vi "Async Test.vi"(11 "gRPCid":T1) -> ()   [LabVIEW 2019]
uses:
  ScanList/labview-grpc-query-server/VIs/MeasurementServer_gRPCid.ctl
  ScanList/labview-grpc-query-server/VIs/MeasurementServer_ErrorOutData.ctl
  ScanList/labview-grpc-query-server/VIs/MeasurementServer_FourProbeRawData.ctl
  ScanList/labview-grpc-query-server/VIs/labview-grpc-measurement-server.lvlib
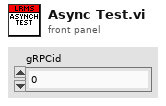
[diagram p1: front panel]
types:
  T1 = typedef "labview-grpc-measurement-server.lvlib/MeasurementServer_gRPCid.ctl" = u64
  T2 = typedef "labview-grpc-measurement-server.lvlib/MeasurementServer_FourProbeRawData.ctl" = cluster{"Positive Voltage":dbl, "Positive Current":dbl, "Negative Voltage":dbl, "Negative Current":dbl, "Impedance":dbl, "ErrorOutData":T3}
  T3 = typedef "labview-grpc-measurement-server.lvlib/MeasurementServer_ErrorOutData.ctl" = cluster{"ErrorCode":i32, "ErrorMessage":string}
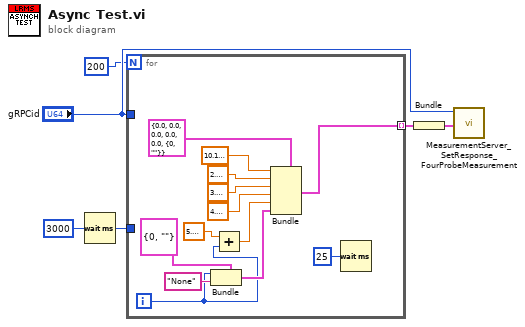
[diagram p0: block diagram]
diagram:
  n1 = Wait (ms)(milliseconds to wait=u32 3000) -> (millisecond timer value=w2:u32)
  n2 = for {
    N: 200 -> [_]
    tunnel: w2 -> [_]
    tunnel: "gRPCid" -> [_]
    tunnel: [w8] -> w5 mode=indexing
    i -> [w11]
    n3 = Bundle(cluster=T3 {"ErrorCode"=0, "ErrorMessage"=""} ("ErrorOutData"), "ErrorCode"=w11, "ErrorMessage"="None") -> (w19:T3)
    n4 = Add(x=sgl 5.1 ("Positive Voltage"), y=w11) -> (x+y=w10:sgl)
    n5 = Bundle(cluster=T2 {"Positive Voltage"=0.0, "Positive Current"=0.0, "Negative Voltage"=0.0, "Negative Current"=0.0, "Impedance"=0.0, "ErrorOutData"={"ErrorCode"=0, "ErrorMessage"=""}} ("FourProbeRawData"), "Positive Voltage"=sgl 10.1, "Positive Current"=sgl 2.1 ("Positive Voltage"), "Negative Voltage"=sgl 3.1 ("Positive Voltage"), "Negative Current"=sgl 4.1 ("Positive Voltage"), "Impedance"=w10, "ErrorOutData"=w19) -> (w8:T2)
    n6 = Wait (ms)(milliseconds to wait=u32 25) -> ()  [unwired: 1 out]
  }
  n7 = Bundle(w5) -> (w6:cluster{T2[]})  [unwired: 1 in]
  n8 = call "MeasurementServer_SetResponse_FourProbeMeasurement.vi"("gRPCid"="gRPCid", "FourProbeResponse"=w6) -> ()  [unwired: 8 in, 1 out]
